vi "Temperature Monitor.vi"() -> ()   [LabVIEW 2015]
doc: "This VI is the solution to an exercise in the LabVIEW Core 1 course.\n\nIt uses a While Loop and shift registers to average data. No hardware is necessary."
panel:
  in  "Stop Button":bool
  out "Temperature History":cluster{dbl, "Temperature Value":dbl}(graph)
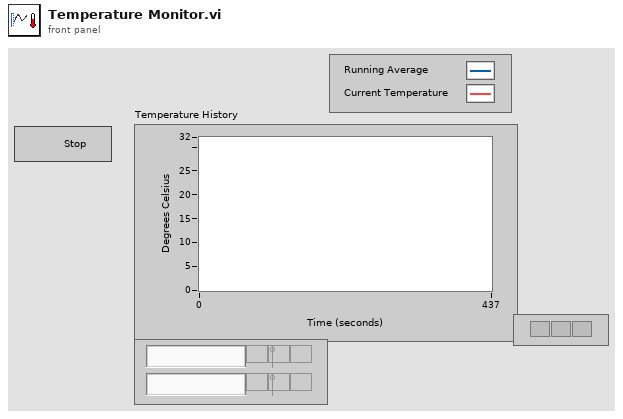
[diagram p1: front panel]
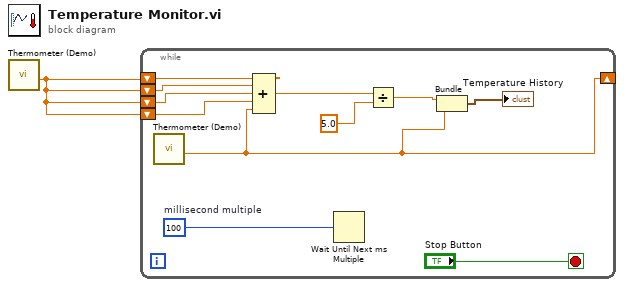
[diagram p0: block diagram]
diagram:
  n1 = call "Thermometer (Demo).vi"() -> ("Temperature Value"=w1:dbl)  [unwired: 11 in]
  n2 = while {
    shift-right: [w4] -> _
    shift-left: w1 -> [w7]
    shift-left: w1 -> [w10]
    shift-left: w1 -> [w9]
    shift-left: w1 -> [w8]
    stop <- "Stop Button" stop-if-true
    w12 = u32 100  # millisecond multiple
    n3 = call "Thermometer (Demo).vi"() -> ("Temperature Value"=w4:dbl)  [unwired: 11 in]
    n4 = Compound Arithmetic op=ADD(w7, w10, w9, w8, w4) -> (w5:dbl)
    n5 = Wait Until Next ms Multiple(millisecond multiple=w12) -> ()  [unwired: 1 out]
    n6 = Divide(x=w5, y=5.0) -> (x/y=w3:dbl)
    n7 = Bundle(w3, "Temperature Value"=w4) -> (→"Temperature History":cluster{dbl, "Temperature Value":dbl})  [unwired: 1 in]
  }
